vi "ReceiveSetDigitalPWMCommand.vi"(0 "Connexion réseau UDP en entrée":refnum<k16>, 1 "entrée d'erreur (pas d'erreur)":errorcluster) -> (2 "Connexion réseau UDP en sortie":refnum<k16>, 3 "sortie d'erreur":errorcluster, 4 "Response Command":u8[](array[numeric]), 5 "Value":u8)   [LabVIEW 2021]
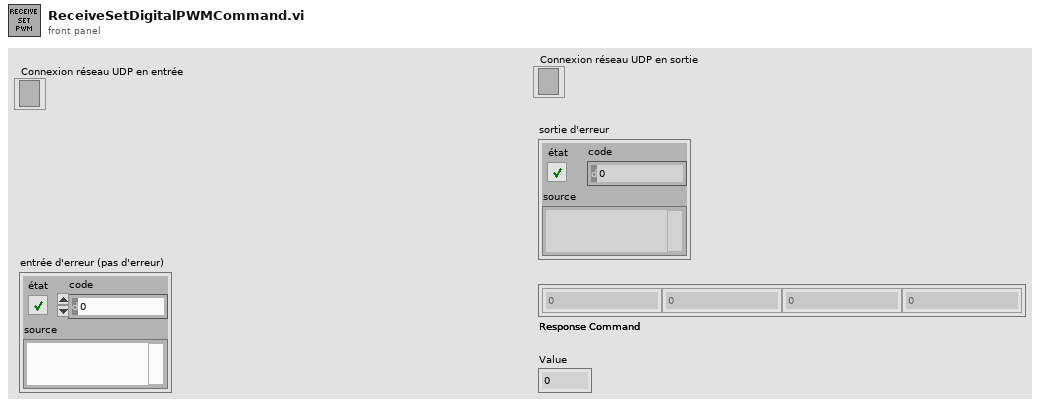
[diagram p1: front panel]
types:
  T1 = typedef "CommandType.ctl" = u8[]
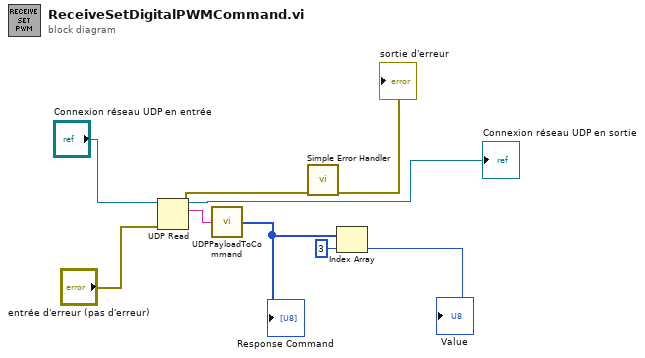
[diagram p0: block diagram]
diagram:
  n1 = UDP Read(connection ID="Connexion réseau UDP en entrée", 8:"entrée d'erreur (pas d'erreur)") -> (data out=w5:string, error out=w6:errorcluster, 3:→"Connexion réseau UDP en sortie":refnum<k16>)  [unwired: 2 in, 2 out]
  n2 = call "UDPPayloadToCommand.vi"("UDP Payload"=w5) -> ("Command"=w2:T1)
  "Response Command" <- w2
  n3 = call <vilib>:"Simple Error Handler.vi"("error in (no error)"=w6) -> ("error out"=→"sortie d'erreur":errorcluster)  [unwired: 4 in, 4 out]
  n4 = Index Array(array=w2, index=3 ("indice")) -> (element=→"Value":u8)
